vi "Load Config INI from File.vi"(6 "File Name":string, 7 "File Type":string(combo)=".gif", 8 "Error In":errorcluster, 10 "reference":refnum<vi>, 11 "Path In":path) -> (0 "Error Out":errorcluster, 3 "Path Out":path)   [LabVIEW 2025]
uses:
  <vilib>/Utility/config.llb/Read Key (String).vi
  <vilib>/Utility/config.llb/NI_LVConfig.lvlib
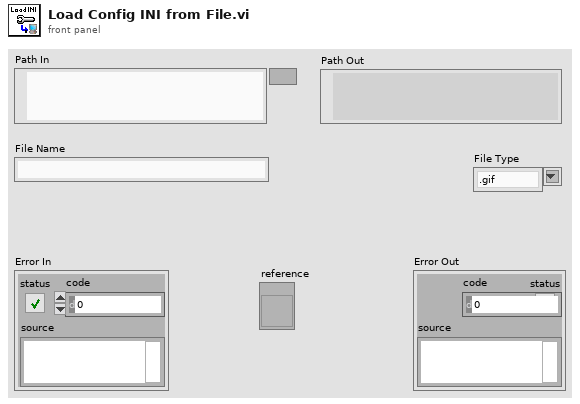
[diagram p1: front panel]
types:
  T1 = typedef "NI_LVConfig.lvlib/Config Data RefNum.ctl" = refnum<k1>
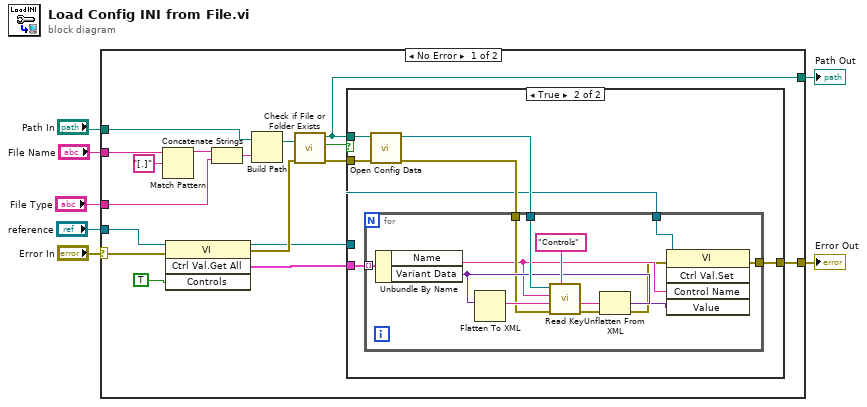
[diagram p0: block diagram]
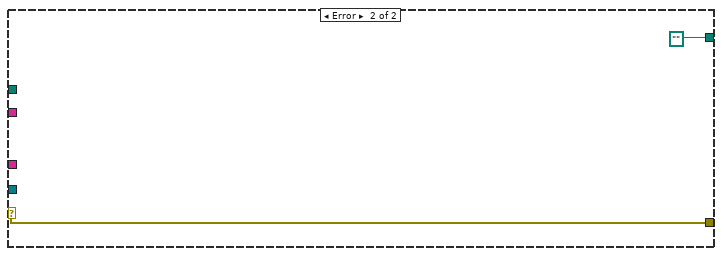
[diagram p3: hidden frame]
diagram:
  n1 = case shown="No Error" "Error In" {
    selector: "Error In" -> [w17 w47]
    tunnel: [w13 w47] -> w5
    tunnel: [w12 path ""] -> w4
    tunnel: "Path In" -> [w9 _]
    tunnel: "reference" -> [w11 _]
    tunnel: "File Type" -> [w10 _]
    tunnel: "File Name" -> [w8 _]
    frame No Error {
      n2 = Match Pattern(string=w8, regular expression="[.]" ("search string")) -> (before substring=w23:string)  [unwired: 1 in, 3 out]
      n3 = invoke class="VI" method="Ctrl Val.Get All"(reference=w11, error in=w17, "Controls"=TRUE) -> (reference out=w14:refnum<vi>, error out=w16:errorcluster, "Get All Control Values Variant"=w15:cluster{"Name":string, "Variant Data":variant}[])  [unwired: 1 in, 1 out]
      n4 = Concatenate Strings(w23, w10) -> (w22:string)
      n5 = Build Path(base path=w9, name or relative path=w22) -> (appended path=w21:path)
      n6 = call <vilib>:"Check if File or Folder Exists.vi"("error in (no error)"=w16, "path"=w21) -> ("error out"=w19:errorcluster, "file or folder exists?"=w20:bool, "dup path"=w12:path)  [unwired: 7 in]
      n7 = case shown="True" w20 {
        tunnel: w12 -> [_ w32]
        tunnel: w19 -> [w25 w31]
        tunnel: w15 -> [_ w30]
        tunnel: w14 -> [_ w27]
        tunnel: [w25 w26] -> w13
        frame False {
        }
        frame True {
          n8 = call <vilib>:"Open Config Data.vi"("error in (no error)"=w31, "configuration file path"=w32) -> ("error out"=w28:errorcluster, "refnum"=w29:T1)  [unwired: 1 in, 7 out]
          n9 = for {
            tunnel: w30 -> [w44] mode=indexing
            tunnel: w29 -> [w43]
            tunnel: w28 -> [w39]
            tunnel: w27 -> [w37]
            tunnel: [w33] -> w26
            n10 = Unbundle By Name(w44) -> ("Name"=w36:string, "Variant Data"=w41:variant)
            n11 = Flatten To XML(6:w41) -> (2:w42:string)
            n12 = call-poly <vilib>:"Read Key.vi"("section"="Controls", "error in (no error)"=w39, "default value"=w42, "key"=w36, "refnum"=w43) -> ("error out"=w38:errorcluster, "value"=w40:string)  [unwired: 3 in, 2 out]
            n13 = Unflatten From XML(xml string=w40, type=w41, error in (no error)=w38) -> (value=w35:variant, error out=w34:errorcluster)
            n14 = invoke class="VI" method="Ctrl Val.Set"(reference=w37, error in=w34, "Control Name"=w36, "Value"=w35) -> (error out=w33:errorcluster)  [unwired: 1 in, 4 out]
          }
        }
      }
    }
    frame Error {
      (unwired) ""
    }
  }
  "Error Out" <- w5
  "Path Out" <- w4
